vi "Teleop.vi"(10 "Match Info":T1={"Autonomous Elapsed Seconds"=0.0, "TeleOp Elapsed Seconds"=0.0, "Disabled Elapsed Seconds"=0.0, "Visited Autonomous"=FALSE, "Visited TeleOp"=FALSE, "Visited Disabled"=FALSE, "Autonomous Settings"={"Autonomous Style"=enum."Independent", "VI Refnum"=refnum}}, 11 "Call Context":T2) -> ()   [LabVIEW 2015]
doc: "This VI is called for each TeleOp packet received from the DS where the robot is not disabled. It is often used to read from the joysticks and update I/O or to update setpoints for timed control loops. It should complete and return within 20 milliseconds or it may miss DS packets."
uses:
  <vilib>/Rock Robotics/WPI/DriverStation/WPI_DriverStationDerivedRobotMode.ctl
  <vilib>/Rock Robotics/WPI/DriverStation/WPI_DriverStationMatch Info.ctl
  <vilib>/Rock Robotics/WPI/Solenoid/WPI_SolenoidValue.ctl
  <vilib>/Rock Robotics/WPI/Utilities/WPI_GetSetVariantRefNum.vi
  <vilib>/Rock Robotics/Network Tables/NT Write Boolean Array.vi
  <vilib>/Rock Robotics/Network Tables/NT Read Boolean.vi
  <vilib>/Rock Robotics/Network Tables/NT Read Number.vi
  <vilib>/Rock Robotics/WPI/Solenoid/WPI_SolenoidSetEnum.vi
  <vilib>/Rock Robotics/Network Tables/NT Write Numeric Array.vi
panel:
  out "Sample Slider 0":dbl(slide) scale=0.0..5.0
  out "Sample Boolean 1":bool
  out "Sample Boolean 0":bool
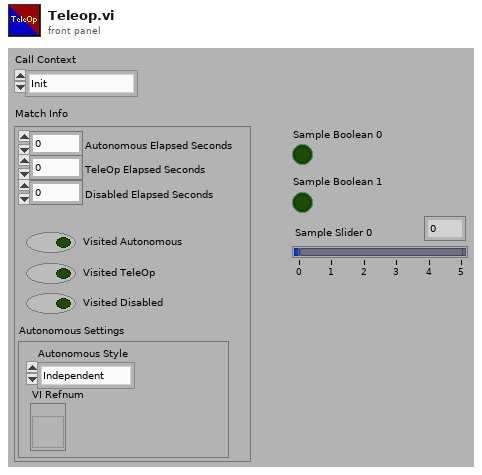
[diagram p1: front panel]
types:
  T1 = typedef "WPI_DriverStationMatch Info.ctl" = cluster{"Autonomous Elapsed Seconds":dbl, "TeleOp Elapsed Seconds":dbl, "Disabled Elapsed Seconds":dbl, "Visited Autonomous":bool, "Visited TeleOp":bool, "Visited Disabled":bool, "Autonomous Settings":cluster{"Autonomous Style":enum16{"Iterative", "Independent"}, "VI Refnum":refnum<vi>}}
  T2 = typedef "WPI_DriverStationDerivedRobotMode.ctl" = enum16{"Init", "Execute", "Stop"}
  T3 = typedef "WPI_SolenoidValue.ctl" = enum16{"Off", "On", "Forward", "Reverse"}
  T4 = typedef "WPI_JoystickDevRef.ctl" = cluster{"Device":T5}
  T5 = typedef "WPI_JoystickDeviceEnum.ctl" = enum16{"USB 0", "USB 1", "USB 2", "USB 3", "USB 4", "USB 5"}
  T6 = typedef "WPI_CompressorDevRef.ctl" = cluster{"DevStatus":errorcluster, "Pneumatics Control Module":u8}
  T7 = typedef "WPI_ServoDeviceRef.ctl" = cluster{"DeviceStatus":errorcluster, "PWM Channel":T8, "DeadBand":T9}
  T8 = typedef "FPGA_DIOPWMChannel.ctl" = enum8{"PWM 0", "PWM 1", "PWM 2", "PWM 3", "PWM 4", "PWM 5", "PWM 6", "PWM 7", "PWM 8", "PWM 9", "PWM MXP 0", "PWM MXP 1", "PWM MXP 2", "PWM MXP 3", "PWM MXP 4", "PWM MXP 5", "PWM MXP 6", "PWM MXP 7", "PWM MXP 8", "PWM MXP 9", "Invalid"}
  T9 = typedef "WPI_PWMDeadband.ctl" = cluster{"Name":string, "maxPositivePwm":i32, "minPositivePwm":i32, "centerPwm":i32, "maxNegativePwm":i32, "minNegativePwm":i32, "angularRange":u16}
  T10 = typedef "WPI_MotorControlDeviceRef.ctl" = cluster{"DeviceStatus":errorcluster, "Type":T11, "PWM":cluster{"PWM Channel":T8, "DeadBand":T9}, "CAN":cluster{"Device Number":u8, "Control Mode":T12, "Semaphore":T13, "Max Vout":dbl, "TalonSRX Control Mode":T14}, "Invert":bool}
  T11 = typedef "WPI_MotorControlType.ctl" = enum16{"PWM", "CAN", "CANTalonSRX"}
  T12 = typedef "WPI_CANJaguar_ControlMode.ctl" = enum8{"Percent VBus", "Current", "Speed", "Position", "Voltage"}
  T13 = typedef "Semaphore RefNum" = refnum<k1>
  T14 = typedef "WPI_CANTalonSRX_APIControlMode.ctl" = enum8{"Percent VBus", "Speed", "Position", "Slave", "Unchanged / Invalid", "Voltage Compensation", "Current", "Motion Profile"}
  T15 = typedef "WPI_DigitalInputDevRef.ctl" = cluster{"DevStatus":errorcluster, "DIO Channel":T16}
  T16 = typedef "FPGA_DIOChannel.ctl" = enum8{"DIO 0", "DIO 1", "DIO 2", "DIO 3", "DIO 4", "DIO 5", "DIO 6", "DIO 7", "DIO 8", "DIO 9", "DIO MXP 0", "DIO MXP 1", "DIO MXP 2", "DIO MXP 3", "DIO MXP 4", "DIO MXP 5", "DIO MXP 6", "DIO MXP 7", "DIO MXP 8", "DIO MXP 9", "DIO MXP 10", "DIO MXP 11", "DIO MXP 12", "DIO MXP 13", "DIO MXP 14", "DIO MXP 15", "Invalid"}
  T17 = typedef "WPI_RobotDriveDevRef.ctl" = cluster{"DevStatus":errorcluster, "Motors[]":T10[], "Square Inputs":bool, "Max Output":dbl}
  T18 = typedef "WPI_SolenoidDevRef.ctl" = cluster{"DevStatus":errorcluster, "Pneumatics Control Module":u8, "Forward Solenoid Channel":T19, "Reverse Solenoid Channel":T19}
  T19 = typedef "WPI_SolenoidChannel.ctl" = enum8{"Solenoid 0", "Solenoid 1", "Solenoid 2", "Solenoid 3", "Solenoid 4", "Solenoid 5", "Solenoid 6", "Solenoid 7", "Invalid"}
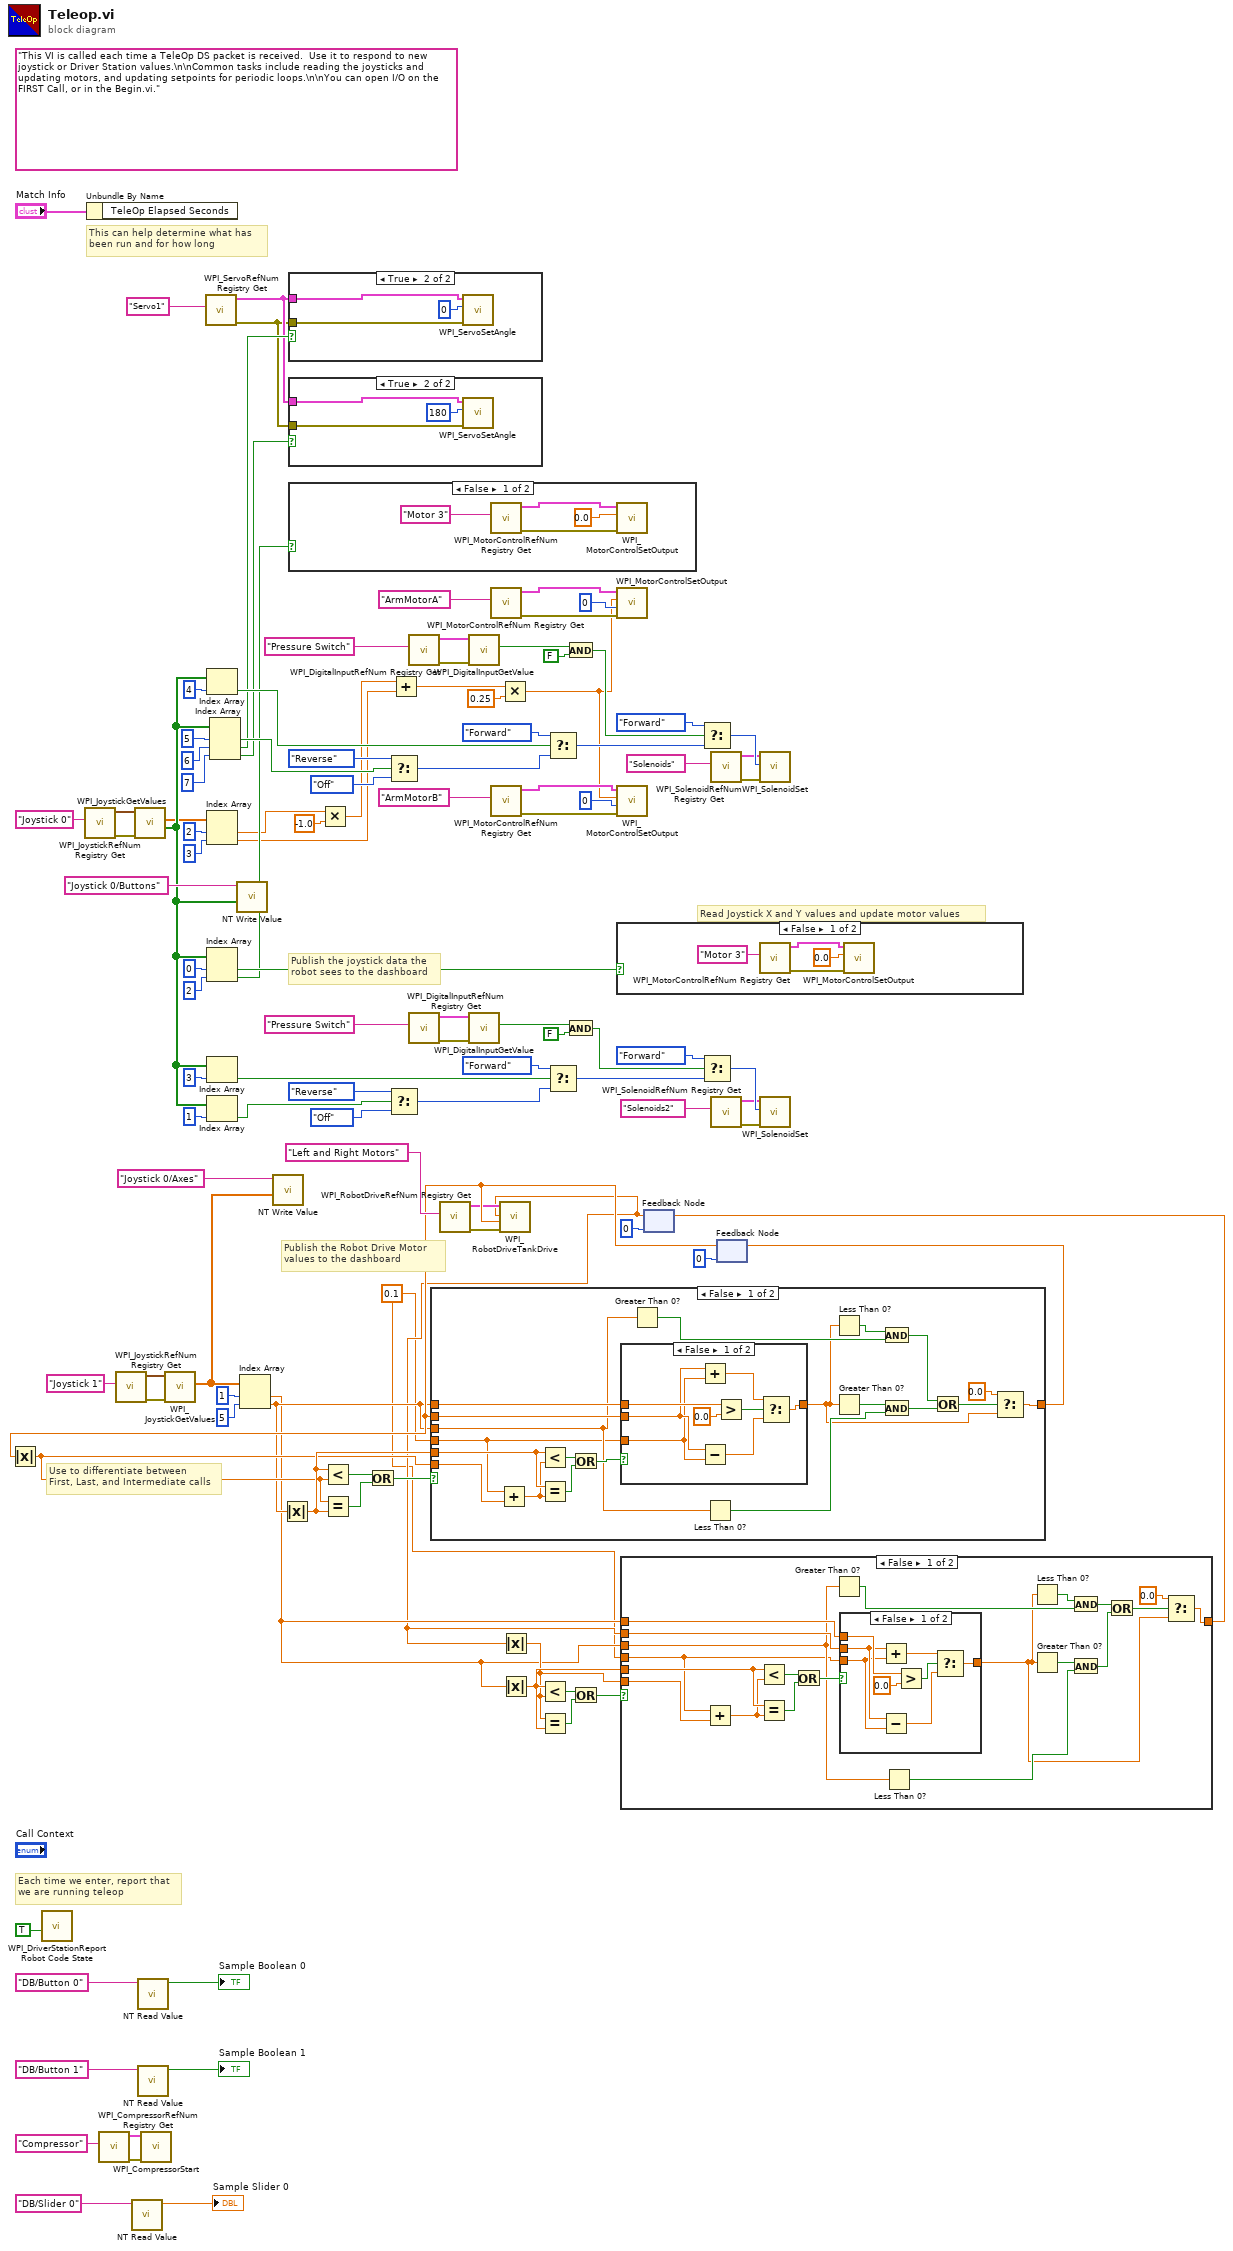
[diagram p0: block diagram]
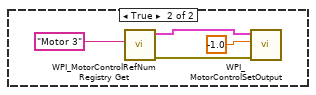
[diagram p8: hidden frame]
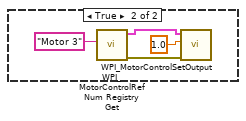
[diagram p9: hidden frame]
diagram:
  w1 = 0.1
  (unwired) "This VI is called each time a TeleOp DS packet is received.  Use it to respond to new joystick or Driver Station values.\n\nCommon tasks include reading the joysticks and updating motors, and updating setpoints for periodic loops.\n\nYou can open I/O on the FIRST Call, or in the Begin.vi."
  # "Publish the Robot Drive Motor\nvalues to the dashboard"
  # "Publish the joystick data the\nrobot sees to the dashboard"
  # "Each time we enter, report that\nwe are running teleop"
  # "Use to differentiate between\nFirst, Last, and Intermediate calls"
  # "This can help determine what has\nbeen run and for how long"
  # "Read Joystick X and Y values and update motor values"
  n1 = call <vilib>:"WPI_DriverStationReport Robot Code State.vi"("TeleOp"=TRUE ("Autonomous")) -> ()  [unwired: 10 in, 1 out]
  n2 = call <vilib>:"WPI_JoystickRefNum Registry Get.vi"("refnum name"="Joystick 0") -> ("error out"=w58:errorcluster, "JoystickDevRef"=w59:T4)  [unwired: 1 in, 8 out]
  n3 = Unbundle By Name("Match Info") -> ()  [unwired: 1 out]
  n4 = call <vilib>:"WPI_CompressorRefNum Registry Get.vi"("refnum name"="Compressor") -> ("error out"=w48:errorcluster, "CompressorDevRef"=w49:T6)  [unwired: 9 in]
  n5 = call <vilib>:"WPI_JoystickRefNum Registry Get.vi"("refnum name"="Joystick 1") -> ("error out"=w52:errorcluster, "JoystickDevRef"=w53:T4)  [unwired: 1 in, 8 out]
  n6 = call-poly <vilib>:"NT Read Value.vi"("Name"="DB/Slider 0" ("refnum name")) -> ("Numeric"=→"Sample Slider 0":dbl)  [unwired: 9 in, 1 out]
  n7 = call <vilib>:"WPI_JoystickGetValues.vi"("error in (no error)"=w58, "JoystickDevRef"=w59) -> ("Buttons"=w45:bool[], "Axes"=w44:dbl[])  [unwired: 5 in, 3 out]
  n8 = call-poly <vilib>:"NT Read Value.vi"("Name"="DB/Button 0" ("refnum name")) -> ("Boolean"=→"Sample Boolean 0":bool)  [unwired: 9 in, 1 out]
  n9 = call-poly <vilib>:"NT Read Value.vi"("Name"="DB/Button 1" ("refnum name")) -> ("Boolean"=→"Sample Boolean 1":bool)  [unwired: 9 in, 1 out]
  n10 = call <vilib>:"WPI_CompressorStart.vi"("error in (no error)"=w48, "CompressorDevRef"=w49) -> ()  [unwired: 8 in, 2 out]
  n11 = call <vilib>:"WPI_JoystickGetValues.vi"("error in (no error)"=w52, "JoystickDevRef"=w53) -> ("Axes"=w56:dbl[])  [unwired: 5 in, 4 out]
  n12 = call <vilib>:"WPI_ServoRefNum Registry Get.vi"("refnum name"="Servo1") -> ("error out"=w13:errorcluster, "ServoDeviceRef"=w14:T7)  [unwired: 9 in]
  n13 = Index Array(array=w45, index=4) -> (element=w87:bool)
  n14 = Index Array(array=w44, index #1=2 ("index"), index #2=3 ("index")) -> (element #1=w41:dbl, element #2=w40:dbl)
  n15 = Index Array(array=w45, index #1=0 ("index"), index #2=2 ("index")) -> (element #1=w55:bool, element #2=w46:bool)
  n16 = Index Array(array=w45, index=3) -> (element=w67:bool)
  n17 = Index Array(array=w45, index=1) -> (element=w73:bool)
  n18 = Index Array(array=w45, index #1=5 ("index"), index #2=6 ("index"), index #3=7 ("index")) -> (element #1=w93:bool, element #2=w16:bool, element #3=w15:bool)
  n19 = call-poly <vilib>:"NT Write Value.vi"("Boolean Array"=w45, "Name"="Joystick 0/Buttons") -> ()  [unwired: 9 in, 1 out]
  n20 = Index Array(array=w56, index #1=1 ("index"), index #2=5 ("index")) -> (element #1=w3:dbl, element #2=w11:dbl)
  n21 = call-poly <vilib>:"NT Write Value.vi"("Numeric Array"=w56, "Name"="Joystick 0/Axes") -> ()  [unwired: 9 in, 1 out]
  n22 = Absolute Value(x=w11) -> (abs(x)=w23:dbl)
  n23 = case shown="True" w16 {
    tunnel: w14 -> [_ w116]
    tunnel: w13 -> [_ w115]
    frame False {
    }
    frame True {
      n24 = call <vilib>:"WPI_ServoSetAngle.vi"("error in (no error)"=w115, "Angle"=0, "ServoDeviceRef"=w116) -> ()  [unwired: 7 in, 2 out]
    }
  }
  n25 = case shown="True" w15 {
    tunnel: w14 -> [_ w119]
    tunnel: w13 -> [_ w118]
    frame False {
    }
    frame True {
      n26 = call <vilib>:"WPI_ServoSetAngle.vi"("error in (no error)"=w118, "Angle"=180, "ServoDeviceRef"=w119) -> ()  [unwired: 7 in, 2 out]
    }
  }
  n27 = case shown="False" w46 {
    frame False {
      n28 = call <vilib>:"WPI_MotorControlRefNum Registry Get.vi"("refnum name"="Motor 3") -> ("error out"=w123:errorcluster, "MotorControlDevRef"=w121:T10)  [unwired: 9 in]
      n29 = call <vilib>:"WPI_MotorControlSetOutput.vi"("error in (no error)"=w123, "Output"=0.0, "MotorControlDevRef"=w121) -> ()  [unwired: 6 in, 3 out]
    }
    frame True {
      n30 = call <vilib>:"WPI_MotorControlRefNum Registry Get.vi"("refnum name"="Motor 3") -> ("error out"=w126:errorcluster, "MotorControlDevRef"=w127:T10)  [unwired: 9 in]
      n31 = call <vilib>:"WPI_MotorControlSetOutput.vi"("error in (no error)"=w126, "Output"=-1.0, "MotorControlDevRef"=w127) -> ()  [unwired: 6 in, 3 out]
    }
  }
  n32 = Multiply(x=w41, y=-1.0) -> (x*y=w50:dbl)
  n33 = Select(t=WPI_SolenoidValue."Reverse" ("Value"), s=w93, f=WPI_SolenoidValue."Off" ("Value")) -> (s? t:f=w88:T3)
  n34 = Select(t=WPI_SolenoidValue."Reverse" ("Value"), s=w73, f=WPI_SolenoidValue."Off" ("Value")) -> (s? t:f=w68:T3)
  n35 = Add(x=w50, y=w40) -> (x+y=w28:dbl)
  n36 = call <vilib>:"WPI_DigitalInputRefNum Registry Get.vi"("refnum name"="Pressure Switch") -> ("error out"=w98:errorcluster, "DigitalInputDevRef"=w97:T15)  [unwired: 9 in]
  n37 = call <vilib>:"WPI_DigitalInputRefNum Registry Get.vi"("refnum name"="Pressure Switch") -> ("error out"=w78:errorcluster, "DigitalInputDevRef"=w77:T15)  [unwired: 9 in]
  n38 = call <vilib>:"WPI_RobotDriveRefNum Registry Get.vi"("refnum name"="Left and Right Motors") -> ("error out"=w39:errorcluster, "RobotDriveDevRef"=w12:T17)  [unwired: 1 in, 8 out]
  n39 = call <vilib>:"WPI_DigitalInputGetValue.vi"("error in (no error)"=w98, "DigitalInputDevRef"=w97) -> ("Value"=w92:bool)  [unwired: 7 in, 2 out]
  n40 = call <vilib>:"WPI_DigitalInputGetValue.vi"("error in (no error)"=w78, "DigitalInputDevRef"=w77) -> ("Value"=w72:bool)  [unwired: 7 in, 2 out]
  n41 = call <vilib>:"WPI_MotorControlRefNum Registry Get.vi"("refnum name"="ArmMotorA") -> ("error out"=w34:errorcluster, "MotorControlDevRef"=w33:T10)  [unwired: 9 in]
  n42 = call <vilib>:"WPI_MotorControlRefNum Registry Get.vi"("refnum name"="ArmMotorB") -> ("error out"=w35:errorcluster, "MotorControlDevRef"=w36:T10)  [unwired: 9 in]
  n43 = Multiply(x=w28, y=0.25) -> (x*y=w30:dbl)
  n44 = Absolute Value(x=w3) -> (abs(x)=w6:dbl)
  n45 = Select(t=WPI_SolenoidValue."Forward" ("Value"), s=w87, f=w88) -> (s? t:f=w82:T3)
  n46 = Select(t=WPI_SolenoidValue."Forward" ("Value"), s=w67, f=w68) -> (s? t:f=w62:T3)
  n47 = And(x=w92, y=FALSE) -> (x .and. y?=w90:bool)
  n48 = And(x=w72, y=FALSE) -> (x .and. y?=w70:bool)
  n49 = call <vilib>:"WPI_MotorControlSetOutput.vi"("error in (no error)"=w34, "Sync Group / Parameter Slot"=u8 0 ("Master Device Number"), "Output"=w30, "MotorControlDevRef"=w33) -> ()  [unwired: 5 in, 3 out]
  n50 = call <vilib>:"WPI_MotorControlSetOutput.vi"("error in (no error)"=w35, "Sync Group / Parameter Slot"=u8 0 ("Master Device Number"), "Output"=w30, "MotorControlDevRef"=w36) -> ()  [unwired: 5 in, 3 out]
  n51 = case shown="False" w55 {
    frame False {
      n52 = call <vilib>:"WPI_MotorControlRefNum Registry Get.vi"("refnum name"="Motor 3") -> ("error out"=w131:errorcluster, "MotorControlDevRef"=w129:T10)  [unwired: 9 in]
      n53 = call <vilib>:"WPI_MotorControlSetOutput.vi"("error in (no error)"=w131, "Output"=0.0, "MotorControlDevRef"=w129) -> ()  [unwired: 6 in, 3 out]
    }
    frame True {
      n54 = call <vilib>:"WPI_MotorControlRefNum Registry Get.vi"("refnum name"="Motor 3") -> ("error out"=w134:errorcluster, "MotorControlDevRef"=w135:T10)  [unwired: 9 in]
      n55 = call <vilib>:"WPI_MotorControlSetOutput.vi"("error in (no error)"=w134, "Output"=1.0, "MotorControlDevRef"=w135) -> ()  [unwired: 6 in, 3 out]
    }
  }
  n56 = feedback #1(0) -> (w2:dbl)
  n57 = Absolute Value(x=w2) -> (abs(x)=w5:dbl)
  n58 = Less?(x=w6, y=w5) -> (x < y?=w9:bool)
  n59 = Equal?(x=w5, y=w6) -> (x = y?=w8:bool)
  n60 = Or(x=w9, y=w8) -> (x .or. y?=w7:bool)
  n61 = case shown="False" w7 {
    tunnel: w6 -> [w156 _]
    tunnel: w5 -> [w155 _]
    tunnel: w3 -> [w152 w166]
    tunnel: [w138 w166] -> w4
    tunnel: w2 -> [w151 _]
    tunnel: w3 -> [w142 _]
    tunnel: w1 -> [w137 _]
    frame False {
      n62 = Add(x=w137, y=w155) -> (x+y=w150:dbl)
      n63 = Less?(x=w156, y=w150) -> (x < y?=w154:bool)
      n64 = Equal?(x=w156, y=w150) -> (x = y?=w153:bool)
      n65 = Or(x=w154, y=w153) -> (x .or. y?=w149:bool)
      n66 = Greater Than 0?(x=w142) -> (x > 0?=w144:bool)
      n67 = case shown="False" w149 {
        tunnel: w152 -> [w162 w165]
        tunnel: [w164 w165] -> w139
        tunnel: w151 -> [w158 _]
        tunnel: w137 -> [w157 _]
        frame False {
          n68 = Add(x=w158, y=w157) -> (x+y=w159:dbl)
          n69 = Subtract(x=w158, y=w157) -> (x-y=w160:dbl)
          n70 = Greater?(x=w162, y=0.0) -> (0:w163:bool)
          n71 = Select(t=w159, s=w163, f=w160) -> (s? t:f=w164:dbl)
        }
        frame True {
        }
      }
      n72 = Less Than 0?(x=w142) -> (x < 0?=w148:bool)
      n73 = Less Than 0?(x=w139) -> (x < 0?=w143:bool)
      n74 = Greater Than 0?(x=w139) -> (x > 0?=w147:bool)
      n75 = And(x=w143, y=w144) -> (x .and. y?=w145:bool)
      n76 = And(x=w147, y=w148) -> (x .and. y?=w146:bool)
      n77 = Or(x=w145, y=w146) -> (x .or. y?=w141:bool)
      n78 = Select(t=0.0, s=w141, f=w139) -> (s? t:f=w138:dbl)
    }
    frame True {
    }
  }
  n79 = feedback-in #1(w4) -> ()
  n80 = Select(t=WPI_SolenoidValue."Forward" ("Value"), s=w90, f=w82) -> (s? t:f=w85:T3)
  n81 = Select(t=WPI_SolenoidValue."Forward" ("Value"), s=w70, f=w62) -> (s? t:f=w65:T3)
  n82 = call <vilib>:"WPI_SolenoidRefNum Registry Get.vi"("refnum name"="Solenoids") -> ("error out"=w83:errorcluster, "SolenoidDevRef"=w84:T18)  [unwired: 9 in]
  n83 = call <vilib>:"WPI_SolenoidRefNum Registry Get.vi"("refnum name"="Solenoids2") -> ("error out"=w63:errorcluster, "SolenoidDevRef"=w64:T18)  [unwired: 9 in]
  n84 = feedback #2(0) -> (w20:dbl)
  n85 = Absolute Value(x=w20) -> (abs(x)=w22:dbl)
  n86 = Less?(x=w23, y=w22) -> (x < y?=w26:bool)
  n87 = Equal?(x=w22, y=w23) -> (x = y?=w25:bool)
  n88 = Or(x=w26, y=w25) -> (x .or. y?=w24:bool)
  n89 = case shown="False" w24 {
    tunnel: w23 -> [w186 _]
    tunnel: w22 -> [w185 _]
    tunnel: w11 -> [w182 w196]
    tunnel: [w168 w196] -> w21
    tunnel: w20 -> [w181 _]
    tunnel: w11 -> [w172 _]
    tunnel: w1 -> [w167 _]
    frame False {
      n90 = Add(x=w167, y=w185) -> (x+y=w180:dbl)
      n91 = Less?(x=w186, y=w180) -> (x < y?=w184:bool)
      n92 = Equal?(x=w186, y=w180) -> (x = y?=w183:bool)
      n93 = Or(x=w184, y=w183) -> (x .or. y?=w179:bool)
      n94 = case shown="False" w179 {
        tunnel: w182 -> [w192 w195]
        tunnel: [w194 w195] -> w169
        tunnel: w181 -> [w188 _]
        tunnel: w167 -> [w187 _]
        frame False {
          n95 = Add(x=w188, y=w187) -> (x+y=w189:dbl)
          n96 = Subtract(x=w188, y=w187) -> (x-y=w190:dbl)
          n97 = Greater?(x=w192, y=0.0) -> (0:w193:bool)
          n98 = Select(t=w189, s=w193, f=w190) -> (s? t:f=w194:dbl)
        }
        frame True {
        }
      }
      n99 = Greater Than 0?(x=w172) -> (x > 0?=w174:bool)
      n100 = Less Than 0?(x=w172) -> (x < 0?=w178:bool)
      n101 = Less Than 0?(x=w169) -> (x < 0?=w173:bool)
      n102 = Greater Than 0?(x=w169) -> (x > 0?=w177:bool)
      n103 = And(x=w173, y=w174) -> (x .and. y?=w175:bool)
      n104 = And(x=w177, y=w178) -> (x .and. y?=w176:bool)
      n105 = Or(x=w175, y=w176) -> (x .or. y?=w171:bool)
      n106 = Select(t=0.0, s=w171, f=w169) -> (s? t:f=w168:dbl)
    }
    frame True {
    }
  }
  n107 = call <vilib>:"WPI_RobotDriveTankDrive.vi"("error in (no error)"=w39, "Right axis value"=w20, "Left axis value"=w2, "RobotDriveDevRef 2"=w12) -> ()  [unwired: 5 in, 3 out]
  n108 = feedback-in #2(w21) -> ()
  n109 = call-poly <vilib>:"WPI_SolenoidSet.vi"("error in (no error)"=w83, "Value"=w85, "SolenoidDevRef"=w84) -> ()  [unwired: 7 in, 2 out]
  n110 = call-poly <vilib>:"WPI_SolenoidSet.vi"("error in (no error)"=w63, "Value"=w65, "SolenoidDevRef"=w64) -> ()  [unwired: 7 in, 2 out]
